vi "Lesson1 - Event Structure.vi"() -> ()   [LabVIEW 2013]
uses:
  <vilib>/event_ctls.llb/eventsource.ctl
panel:
  out "Source":T1 items=["LabVIEW UI"=0, "ActiveX"=1, "User Event"=25]
  out "Iteration Counter":i32
  in  "Stop Button":bool
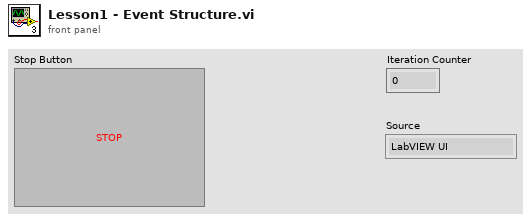
[diagram p1: front panel]
types:
  T1 = typedef "eventsource.ctl" = u32
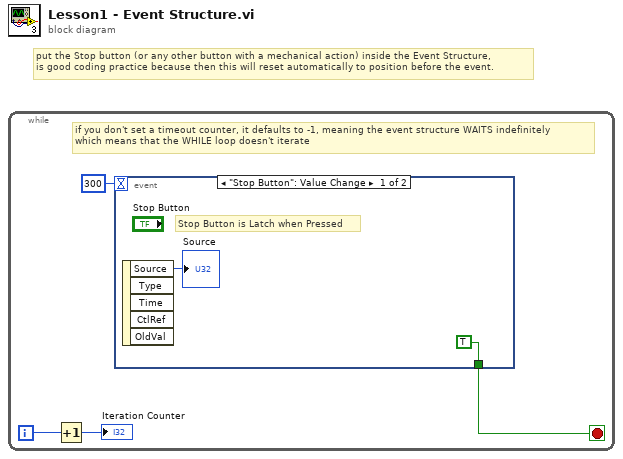
[diagram p0: block diagram]
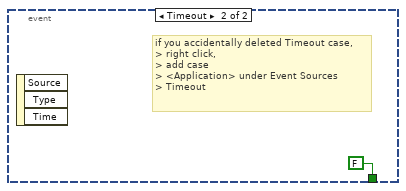
[diagram p2: hidden frame]
diagram:
  # "put the Stop button (or any other button with a mechanical action) inside the Event Structure, \nis good coding practice because then this will reset automatically to position before the event."
  n1 = while {
    i -> [w3]
    stop <- w2 stop-if-true
    # "if you don't set a timeout counter, it defaults to -1, meaning the event structure WAITS indefinitely\nwhich means that the WHILE loop doesn't iterate"
    n2 = Increment(x=w3) -> (x+1=→"Iteration Counter":i32)
    n3 = event shown="[0] \"Stop Button\": Value Change" {
      selector: _ -> [_ _]
      dyn-events: _ -> [_ _]
      timeout: 300 -> [_ _]
      tunnel: [TRUE FALSE] -> w2
      event "Stop Button": Value Change {
        # "Stop Button is Latch when Pressed"
        n4 = event-data() -> ("Source"=→"Source":T1)  [unwired: 1 in, 4 out]
      }
      event Timeout {
        # "if you accidentally deleted Timeout case,\n> right click, \n> add case\n> <Application> under Event Sources\n> Timeout"
        n5 = event-data() -> ()  [unwired: 1 in, 3 out]
      }
    }
  }
